vi "Create Sync Values.vi"() -> ()   [LabVIEW 2018]
doc: "This VI generates 3 random numbers as 64 bit strings. The strings are displayed as Fixed Point numbers that are 38:12 signed values. These random values are used to separate blocks of data as sent from the FPGA to the RT system. The values are stored as constants in the FPGA. The probability that all 3 strings of 38 bits are randomly part of the actual data stream is vanishingly small (38*3 = 114, 2^114 ~ 10^42) or essentially zero.\nAuthor: Scott Hannahs <sth@magnet.fsu.edu>\nCopyright 2018 Florida State University, All rights reserved."
panel:
  out "Raw Hex":u64[](array[numeric])=[4000225541394757851, 1800396117909826064, 15667608548013821775] format="%016x"
  out "FXP":fxp<+/-,38,12>[](array[numeric])=[888.2284999489784, 399.7682446986437, -617.0920498371124] format="%.9g"
  out "FXP 2 Hex":u64[](array[numeric])=[4000225541390073856, 1800396117859368960, 15667608548009836544] format="%016x"
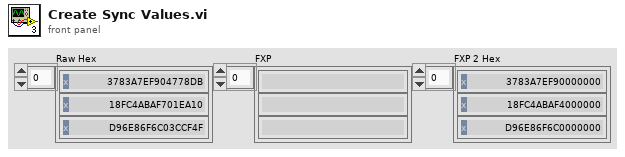
[diagram p1: front panel]
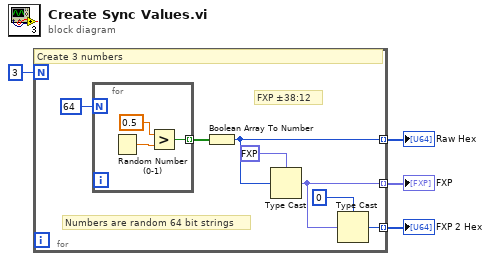
[diagram p0: block diagram]
diagram:
  n1 = for {
    N: 3 -> [_]
    tunnel: [w7] -> w3 mode=indexing
    tunnel: [w6] -> w2 mode=indexing
    tunnel: [w5] -> w1 mode=indexing
    # "FXP ±38:12"
    # "Numbers are random 64 bit strings"
    # "Create 3 numbers"
    n2 = for {
      N: 64 -> [_]
      tunnel: [w13] -> w10 mode=indexing
      n3 = Random Number (0-1)() -> (number: 0 to 1=w14:dbl)
      n4 = Greater?(x=0.5, y=w14) -> (0:w13:bool)
    }
    n5 = Boolean Array To Number(Boolean array=w10) -> (number=w5:u64)
    n6 = Type Cast(type=fxp<+/-,38,12> 0.0 ("Numeric"), x=w5) -> (*(type *) &x=w6:fxp<+/-,38,12>)
    n7 = Type Cast(type=u64 0 ("Numeric 2"), x=w6) -> (*(type *) &x=w7:u64)
  }
  "FXP 2 Hex" <- w3
  "FXP" <- w2
  "Raw Hex" <- w1
